vi "GUI_FilterWheels-BellaAlpha.vi"() -> ()   [LabVIEW 2020]
uses:
  Device Drivers/FilterWheels/posTypDef.ctl
  Device Drivers/FilterWheels/ModeTypDEf.ctl
  <vilib>/Utility/file.llb/Read From Spreadsheet File (string).vi
panel:
  out "reference out":refnum<vi>
  out "#ofChannels":i32
  out "indecator ref array":refnum<vi>[](array[refnum])
  in  "time to wait (TCP) 2":i32=10
  in  "plot":bool=TRUE
  out "ratio(h)":bool
  out "fixsize":bool
  in  "shotnumber":i32
  out "error (h)":bool
  out "Device Name (h)":string="StagingDG645 1"
  in  "Main Tap":T1(tab)
  out "LoadOut":string[][](array[string])
  in  "Path":path=path "H:/data/ECS dumps/FilterWheels"
  in  "ModeAll":T2
  in  "modeArray":T2[](array[typedef])
  out "Status 2":u32[](array[colorbox])
  out "Name":string[](array[string])
  in  "pos":T3[](array[typedef])
  out "device status":string
  out "local Port":u16=65427
  out "port or service name":u16=65426
  out "Remote Host":string="192.168.11.97"
  in  "timeout ms (slow resp)":i32=500
  in  "reset":bool
  out "All Devices (h)":string[](array[string])=["StagingDG645 1", "StagingDG645 2"]
  in  "time to wait (TCP)":i32=10
  out "error out":errorcluster
  out "connections (hidden)":variant[](array[variant])=[variant(refnum<k16> refnum), variant(refnum<k16> refnum)]
  in  "time to wait (main loop)":i32=10
  out "Data String":string="Amplitude.Ch AB,3.000000000000\r\nAmplitude.Ch CD,4.000000000000\r\nAmplitude.Ch EF,4.000000000000\r\nAmplitude.Ch GH,4.000000000000\r\nAmplitude.Ch T0,4.000000000000\r\nDelay.Ch A,0.000000000000\r\nDelay.Ch B,0.030000000000\r\nDelay.Ch C,0.000000000000\r\nDelay.Ch D,0.030000000000\r\nDelay.Ch E,0.000000000000\r\nDelay.Ch F,0.030000000000\r\nDelay.Ch G,0.000000000000\r\nDelay.Ch H,0.030000000000\r\nDelay.Ch T0,0.000000000000\r\nDelay.Ch T1,0.030000\r\nInhibit,Triggers\r\nLinked.Ch A,T0\r\nLinked.Ch B,A\r\nLinked.Ch C,T0\r\nLinked.Ch D,C\r\nLinked.Ch E,T0\r\nLinked.Ch F,E\r\nLinked.Ch G,T0\r\nLinked.Ch H,G\r\nLocalSavingPath,c:\\temp\r\nSave,off\r\nTrigger.ExecuteSingleShot,\r\nTrigger.Level,1.000000\r\nTrigger.Rate,10.000000\r\nTrigger.Source,External rising edges\r\ntimeout,0.000000\r\nPolarity.Ch AB,Positive\r\nPolarity.Ch CD,Positive\r\nPolarity.Ch EF,Positive\r\nPolarity.Ch GH,Positive\r\nPolarity.Ch T0,Positive\r\n"
  in  "Local Saving Path":path
  out "concatenated string":string
  out "subscriberString":string
  out "error message":string
  out "new data":bool
  out "Data Connection out":bool=TRUE
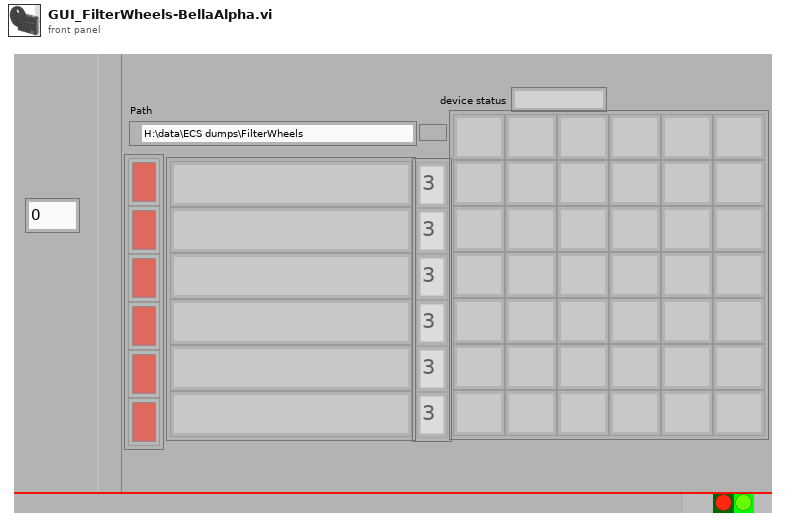
[diagram p1: front panel]
types:
  T1 = enum32{"All Channels", "Network", "Internal", "Advanced"}
  T2 = typedef "ModeTypDEf.ctl" = enum16{"Diode", "Low Power", "High Power", "undefined"}
  T3 = typedef "posTypDef.ctl" = enum16{"1", "2", "3", "4", "5", "6"}
  T4 = typedef "EventTypDef.ctl" = refnum<user-event>
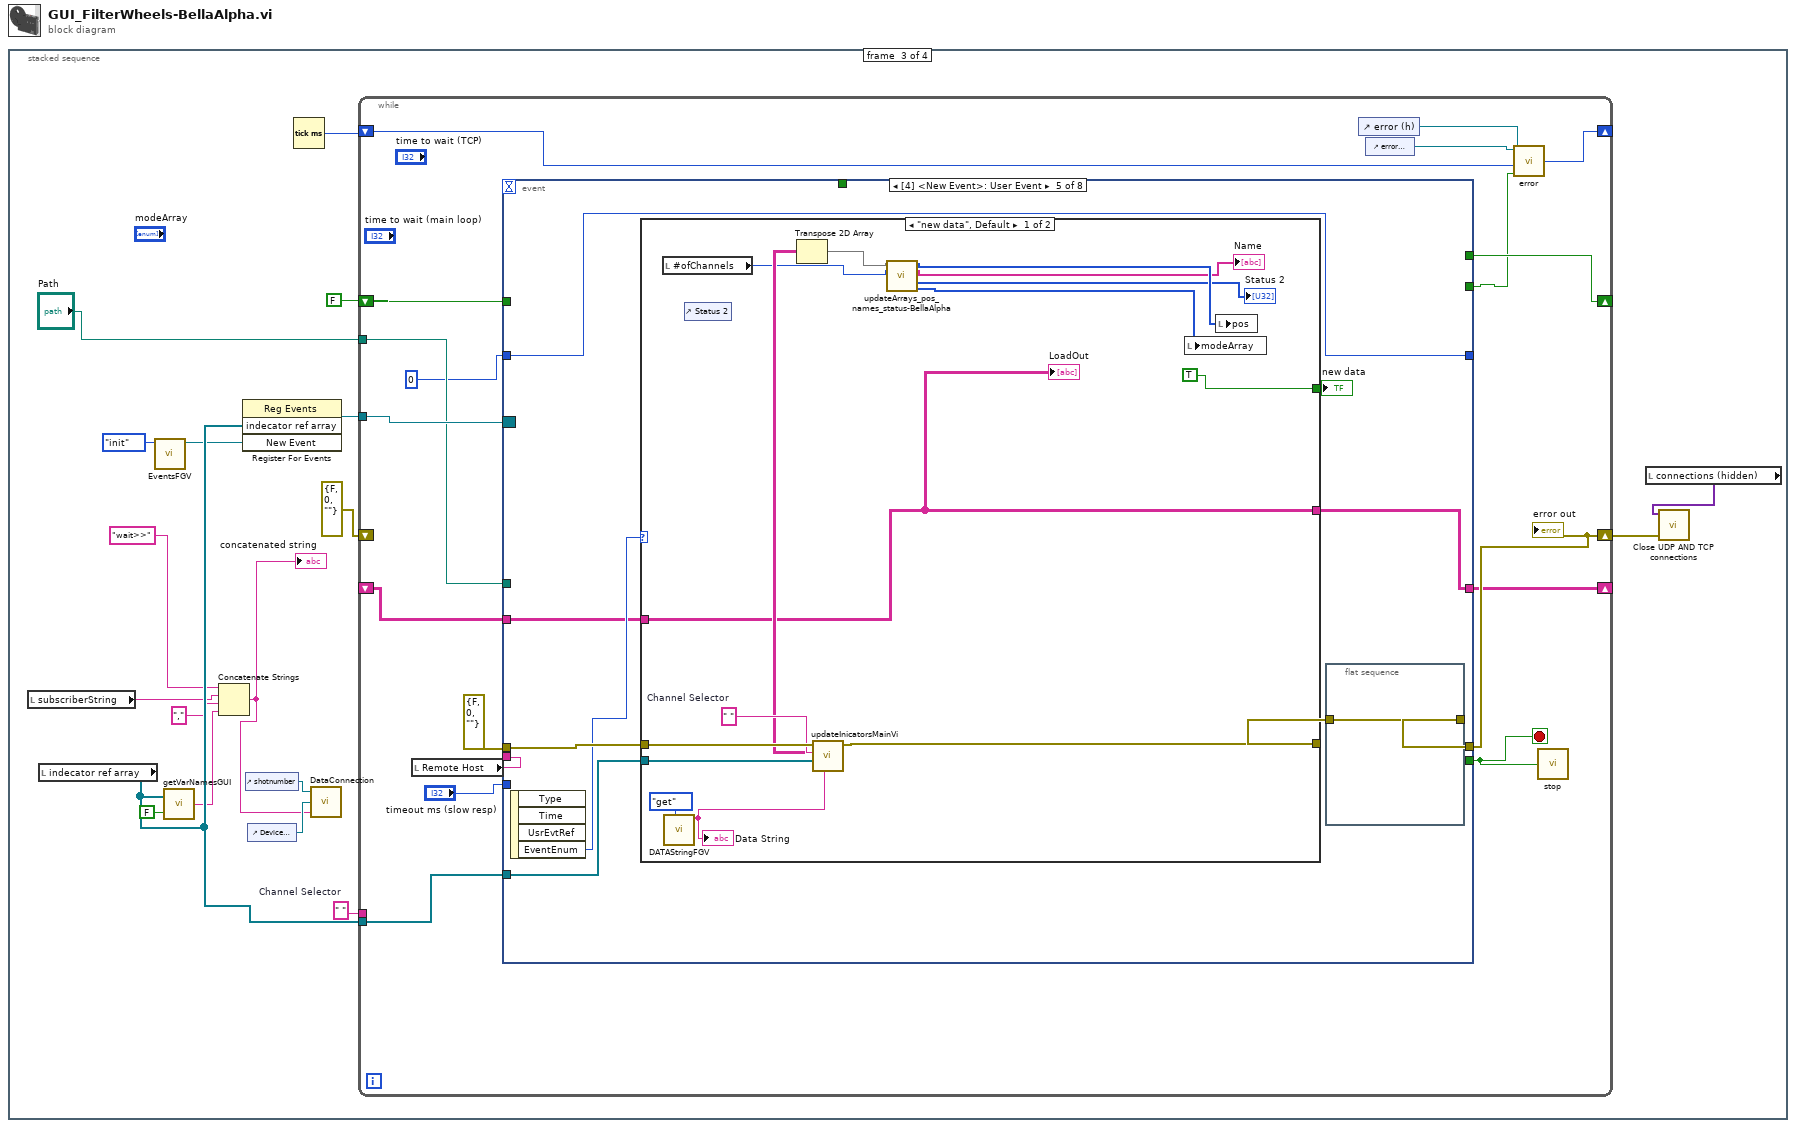
[diagram p0: block diagram]
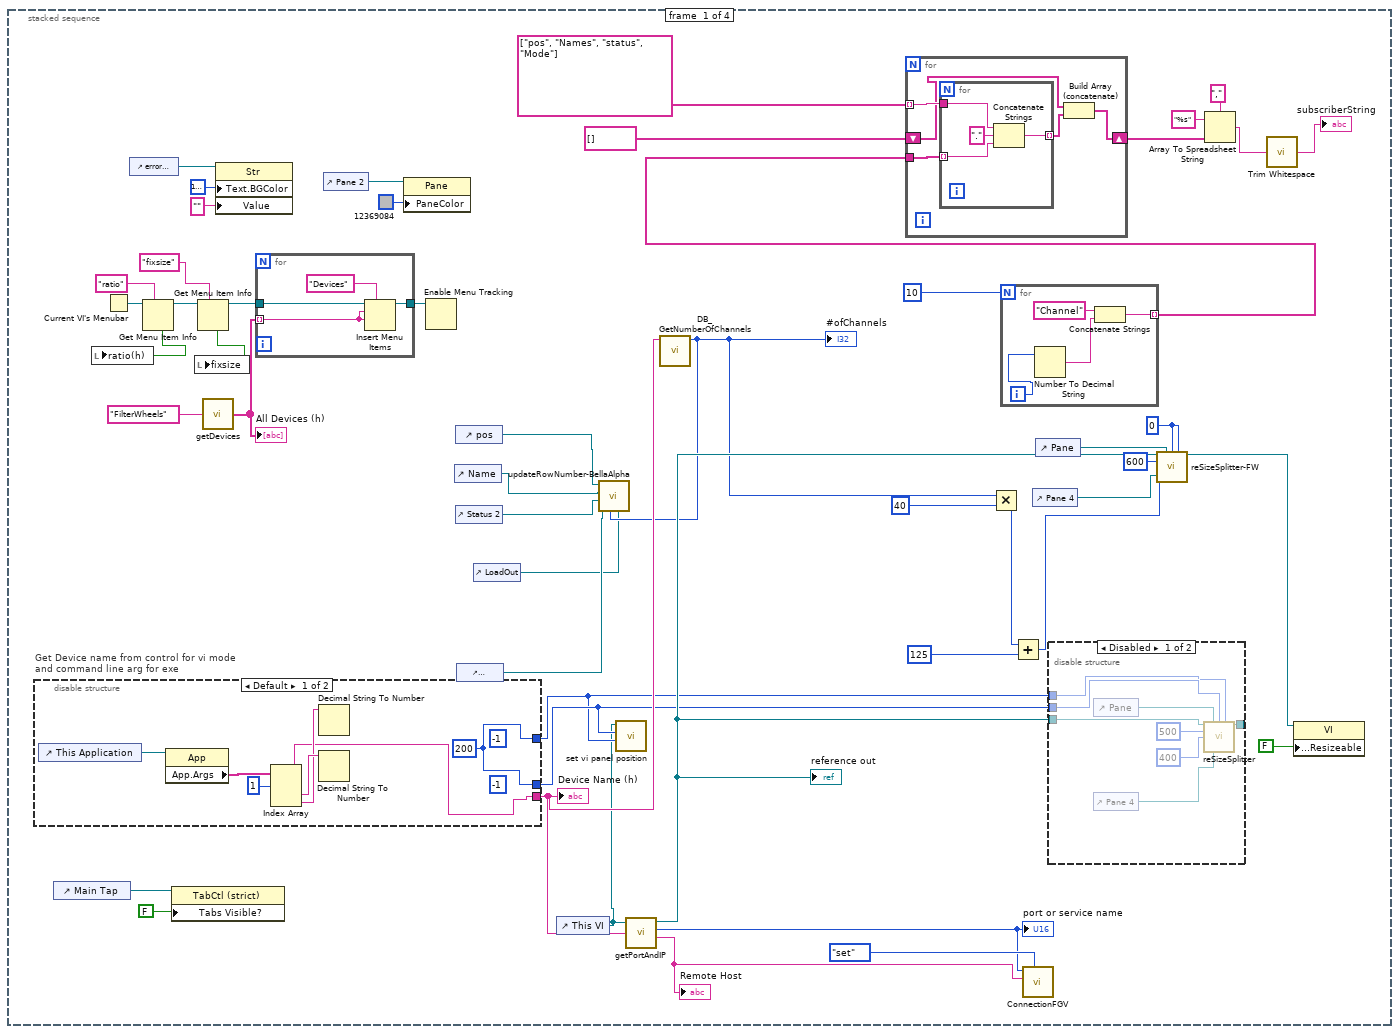
[diagram p2: hidden frame]
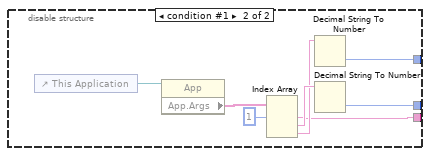
[diagram p4: hidden frame]
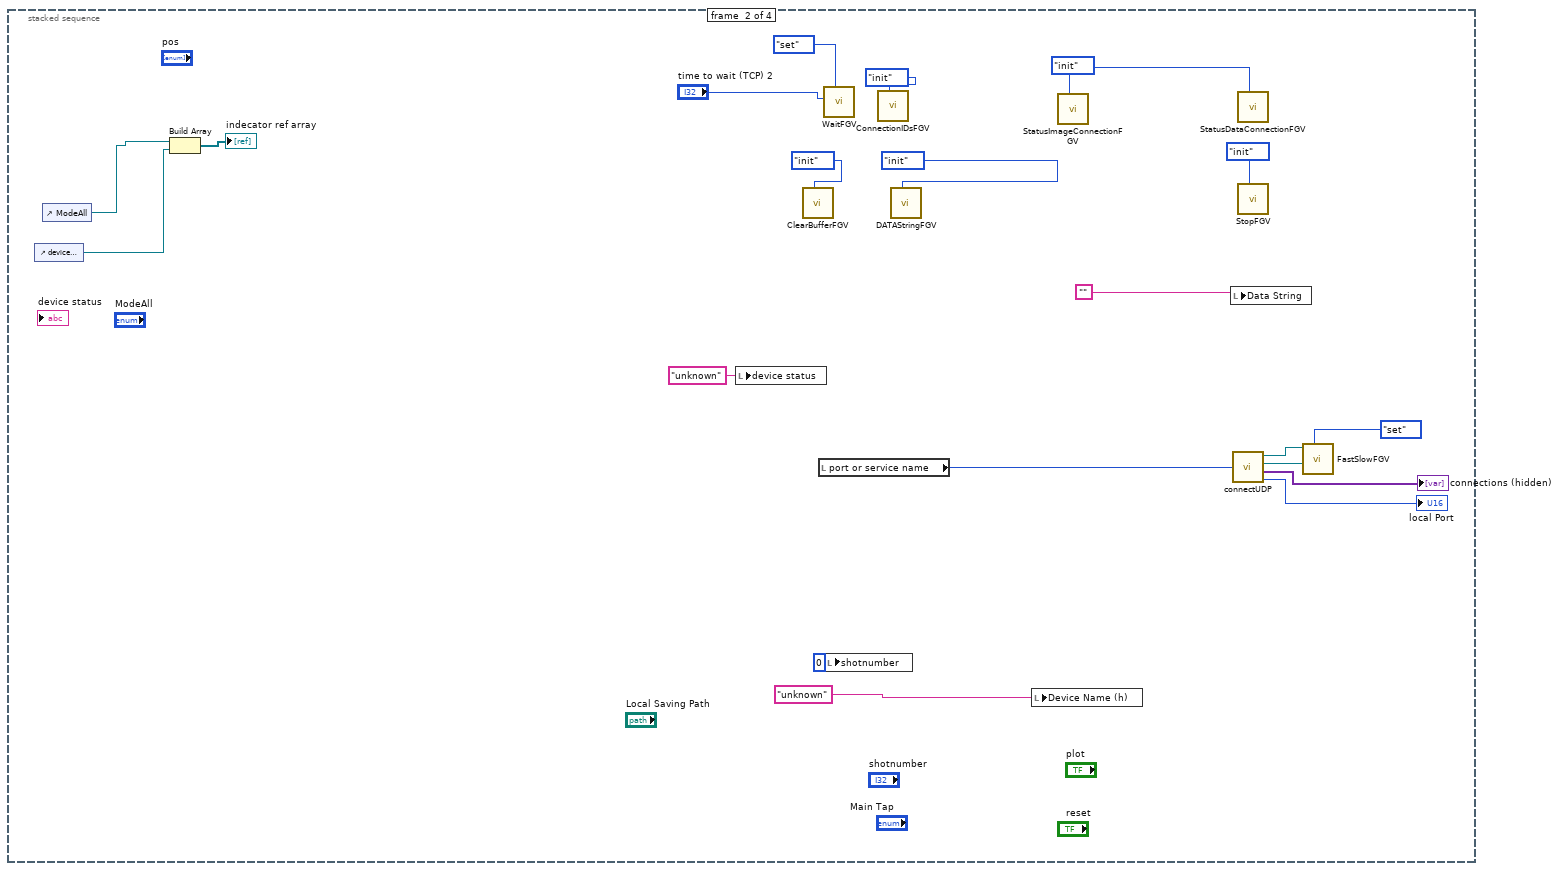
[diagram p5: hidden frame]
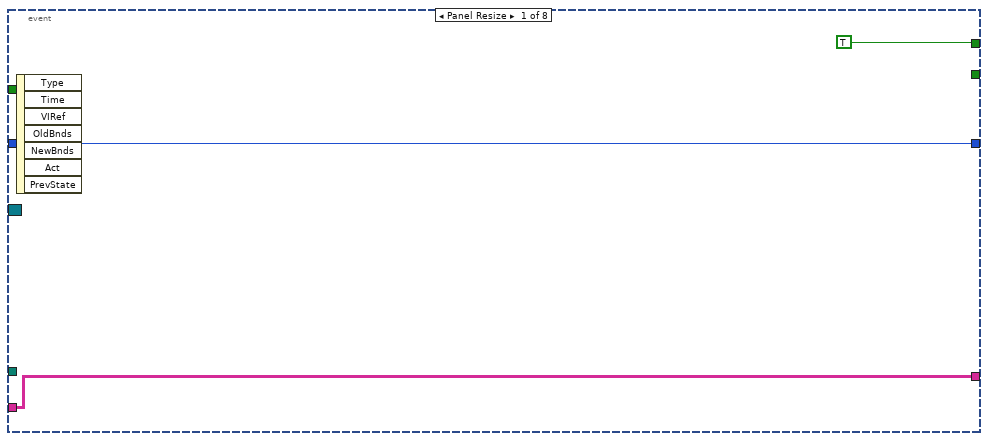
[diagram p6: hidden frame]
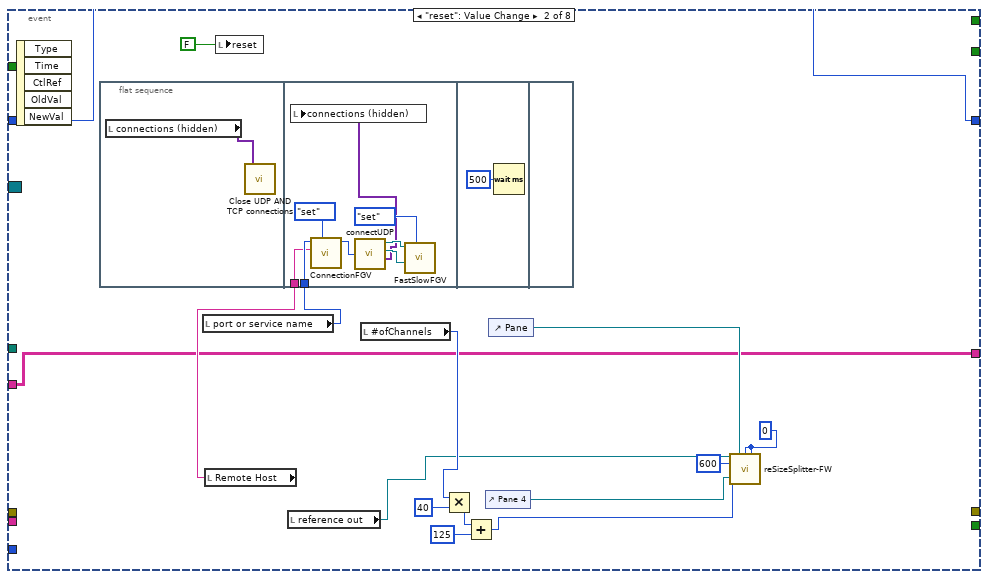
[diagram p7: hidden frame]
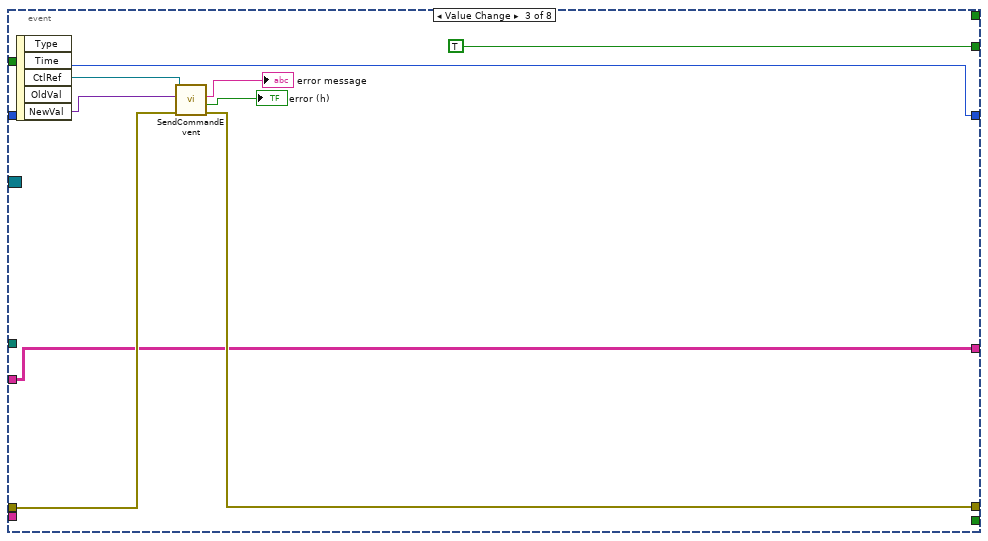
[diagram p8: hidden frame]
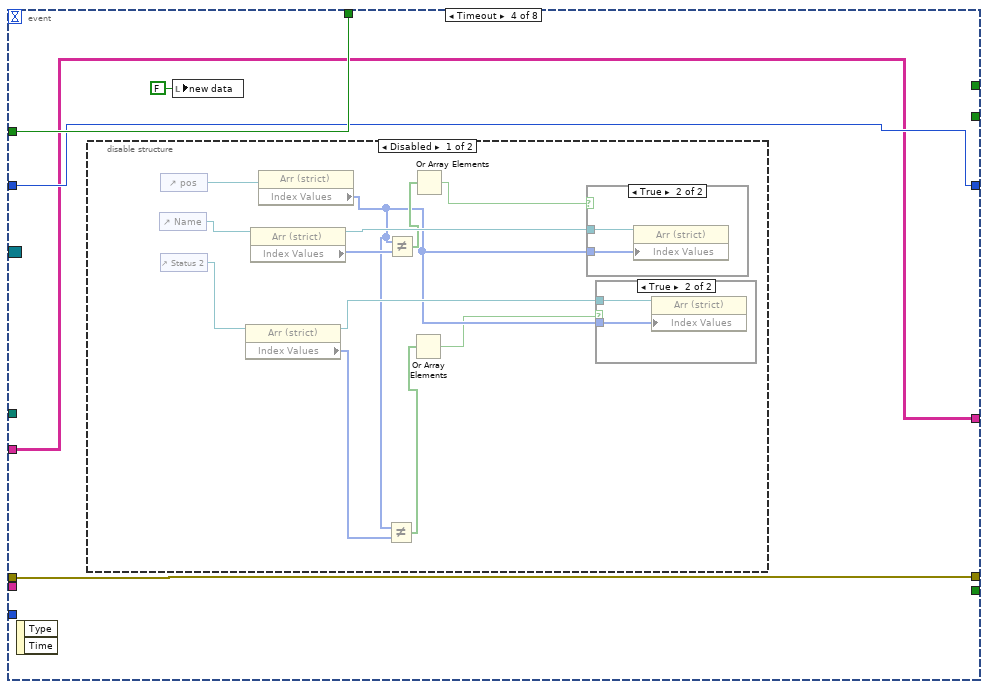
[diagram p9: hidden frame]
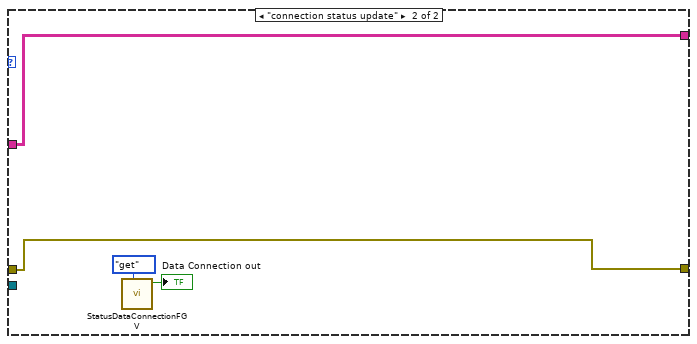
[diagram p13: hidden frame]
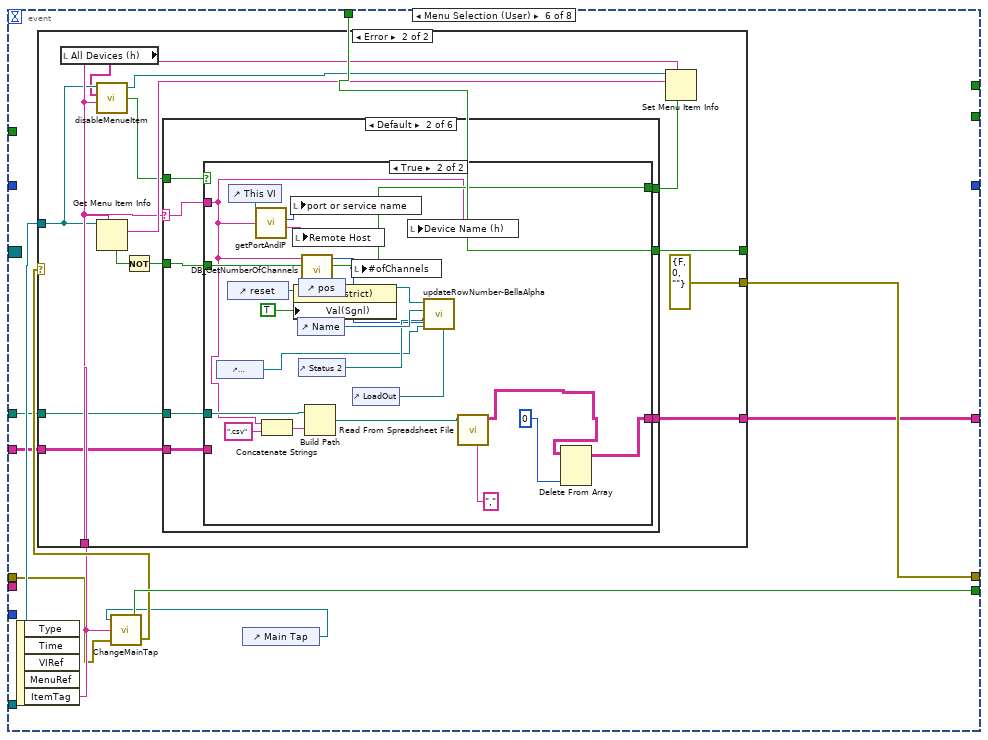
[diagram p14: hidden frame]
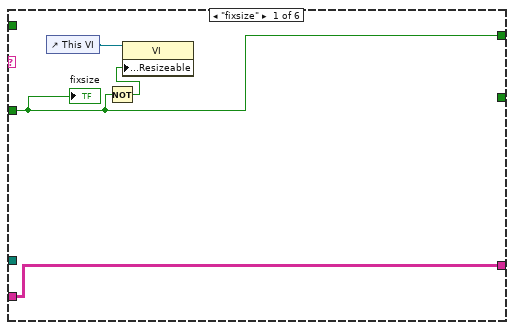
[diagram p16: hidden frame]
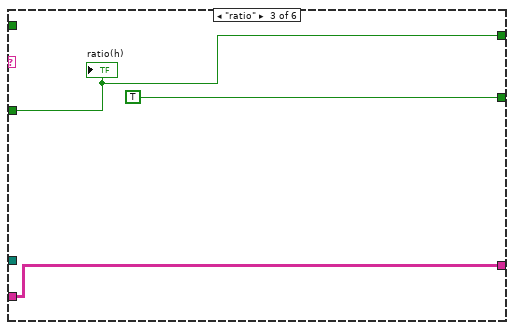
[diagram p18: hidden frame]
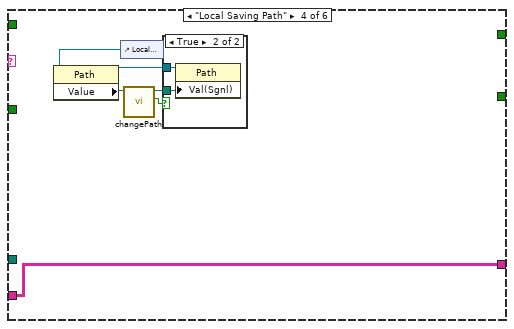
[diagram p19: hidden frame]
diagram:
  n1 = stacked-sequence {
    frame #0 {
      w1 = i16 0 ("top")
      n2 = disable-structure "Get Device name from control for vi mode\nand command line arg for exe" shown="Default" {
        disable-tunnel: [w78 w84] -> w29
        disable-tunnel: [w77 w87] -> w11
        disable-tunnel: [w77 w86] -> w10
        frame condition #0 (active) {
          w77 = i16 200 ("left")
          (unwired) i16 -1 ("left")
          (unwired) i16 -1 ("left")
          n3 = control-ref of="This Application"() -> (w83:refnum<vi>)
          n4 = property class="App"(reference=w83) -> ("App.Args"=w79:string[])  [unwired: 1 in, 2 out]
          n5 = Index Array(array=w79, index #1=1 ("index")) -> (element #1=w78:string, element #2=w81:string, element #3=w80:string)  [unwired: 2 in]
          n6 = Decimal String To Number(string=w80) -> ()  [unwired: 2 in, 2 out]
          n7 = Decimal String To Number(string=w81) -> ()  [unwired: 2 in, 2 out]
        }
        frame condition #1 {
          n8 = control-ref of="This Application"() -> (w91:refnum<vi>)
          n9 = property class="App"(reference=w91) -> ("App.Args"=w85:string[])  [unwired: 1 in, 2 out]
          n10 = Index Array(array=w85, index #1=1 ("index")) -> (element #1=w84:string, element #2=w89:string, element #3=w88:string)  [unwired: 2 in]
          n11 = Decimal String To Number(string=w88) -> (number=w86:i32)  [unwired: 2 in, 1 out]
          n12 = Decimal String To Number(string=w89) -> (number=w87:i32)  [unwired: 2 in, 1 out]
        }
      }
      "Device Name (h)" <- w29
      n13 = control-ref of="Main Tap"() -> (w50:refnum<vi>)
      n14 = Current VI's Menubar() -> (w43:refnum<k9>)
      n15 = control-ref of="error message"() -> (w37:refnum<vi>)
      n16 = Get Menu Item Info(7:"ratio" ("item tag"), 11:w43) -> (3:w41:refnum<k9>, 4:w42:bool)  [unwired: 1 in, 5 out]
      n17 = local write "ratio(h)"(w42) -> ()
      n18 = property class="TabCtl (strict)"(reference=w50, "Tabs Visible?"=FALSE) -> ()  [unwired: 1 in, 2 out]
      n19 = Get Menu Item Info(7:"fixsize" ("item tag"), 11:w41) -> (3:w33:refnum<k9>, 4:w39:bool)  [unwired: 1 in, 5 out]
      n20 = local write "fixsize"(w39) -> ()
      n21 = call "getDevices.vi"("Device Class"="FilterWheels") -> ("All Devices"=w31:string[])
      "All Devices (h)" <- w31
      n22 = property class="Str"(reference=w37, "Text.BGColor"=u32 16777238, "Value"="") -> ()  [unwired: 1 in, 2 out]
      n23 = for {
        tunnel: w33 -> [w67]
        tunnel: [w66] -> w32
        tunnel: w31 -> [w64] mode=indexing
        n24 = Insert Menu Items(5:"Devices" ("menu tag"), 7:w64, 8:w64, 9:w67) -> (3:w66:refnum<k9>)  [unwired: 2 in, 2 out]
      }
      n25 = control-ref of="Pane 2"() -> (w35:refnum<vi>)
      n26 = property class="Pane"(reference=w35, "PaneColor"=u32 12369084) -> ()  [unwired: 1 in, 2 out]
      n27 = Enable Menu Tracking(4:w32) -> ()  [unwired: 2 in, 2 out]
      n28 = control-ref of="Name"() -> (w7:refnum<vi>)
      n29 = control-ref of="pos"() -> (w8:refnum<vi>)
      n30 = control-ref of="Status 2"() -> (w6:refnum<vi>)
      n31 = control-ref of="modeArray"() -> (w5:refnum<vi>)
      n32 = control-ref of="LoadOut"() -> (w3:refnum<vi>)
      n33 = control-ref of="This VI"() -> (w9:refnum<vi>)
      n34 = call "set vi panel position.vi"("top"=w10, "left"=w11, "This VI"=w9) -> ()  [unwired: 7 in, 2 out]
      n35 = call "getPortAndIP.vi"("Device Name"=w29, "This Vi"=w9) -> ("Remote Host"=w46:string, "port or service name"=w45:u16, "reference out"=w18:refnum<vi>)  [unwired: 2 in, 2 out]
      "port or service name" <- w45
      "Remote Host" <- w46
      "reference out" <- w18
      n36 = call "DB_GetNumberOfChannels.vi"("DeviceName"=w29) -> ("Numeric"=w4:i32)  [unwired: 9 in, 1 out]
      "#ofChannels" <- w4
      n37 = call "updateRowNumber-BellaAlpha.vi"("LoadOut"=w3, "Numeric"=w4, "modeArray 2"=w5, "Status 3"=w6, "Name"=w7, "Array in"=w8) -> ()  [unwired: 6 in]
      n38 = Multiply(x=w4, y=40) -> (x*y=w12:i32)
      n39 = for {
        N: 10 -> [_]
        tunnel: [w60] -> w27 mode=indexing
        i -> [w63]
        n40 = Number To Decimal String(number=w63) -> (decimal integer string=w61:string)  [unwired: 1 in]
        n41 = Concatenate Strings("Channel" ("string"), w61) -> (w60:string)
      }
      n42 = for {
        tunnel: string[] ["pos", "Names", "status", "Mode"] -> [w54] mode=indexing
        tunnel: w27 -> [w55]
        shift-right: [w52] -> w24
        shift-left: string[] [] -> [w51]
        n43 = for {
          tunnel: w55 -> [w57] mode=indexing
          tunnel: w54 -> [w59]
          tunnel: [w56] -> w53 mode=indexing
          n44 = Concatenate Strings(w59, "." ("string"), w57) -> (w56:string)
        }
        n45 = Build Array (concatenate)(w51, w53) -> (w52:string[])
      }
      n46 = Add(x=w12, y=125) -> (x+y=w13:i32)
      n47 = call "ConnectionFGV.vi"("command"=enum16{"get", "set", "init"}."set", "Remote Host in"=w46, "port or service name in"=w45) -> ()  [unwired: 7 in, 2 out]
      n48 = control-ref of="Pane 4"() -> (w16:refnum<vi>)
      n49 = control-ref of="Pane"() -> (w19:refnum<vi>)
      n50 = disable-structure shown="Disabled" {
        disable-tunnel: w11 -> [w74 _]
        disable-tunnel: w10 -> [w73 _]
        disable-tunnel: w18 -> [w71 w76]
        disable-tunnel: [w68 w76] -> _
        frame Disabled {
          n51 = control-ref of="Pane"() -> (w75:refnum<vi>)
          n52 = control-ref of="Pane 4"() -> (w72:refnum<vi>)
          n53 = call "reSizeSplitter.vi"("this vi"=w71, "pane"=w75, "left"=w74, "top"=w73, "Width"=u32 500, "Height"=u32 400, "pane2"=w72) -> ("reference out"=w68:refnum<vi>)  [unwired: 8 in]
        }
        frame Enabled {
        }
      }
      n54 = call "reSizeSplitter-FW.vi"("this vi"=w18, "pane"=w19, "left"=w1, "top"=w1, "Width"=u32 600, "Height"=w13, "pane2"=w16) -> ("reference out"=w17:refnum<vi>)  [unwired: 8 in]
      n55 = Array To Spreadsheet String(delimiter (Tab)=",", array=w24, 3:"%s" ("format string")) -> (spreadsheet string=w22:string)
      n56 = call <vilib>:"Trim Whitespace.vi"("string"=w22) -> ("trimmed string"=→"subscriberString":string)  [unwired: 1 in]
      n57 = property class="VI"(reference=w17, "Front Panel.Resizeable"=FALSE ("Front Panel Window:Resizable")) -> ()  [unwired: 1 in, 2 out]
    }
    frame #1 {
      w104 = enum16{"get", "set", "init"}."init" ("Command")
      n58 = control-ref of="device status"() -> (w93:refnum<vi>)
      n59 = control-ref of="ModeAll"() -> (w94:refnum<vi>)
      n60 = Build Array(w94, w93) -> (→"indecator ref array":refnum<vi>[])
      n61 = local write "device status"("unknown" ("device status")) -> ()
      n62 = call "ClearBufferFGV.vi"("Command"=enum16{"set", "get", "init"}."init") -> ()  [unwired: 10 in, 1 out]
      n63 = local read "port or service name"() -> (w100:u16)
      n64 = call "WaitFGV.vi"("Command"=enum16{"get", "set", "init"}."set", "milliseconds to wait"="time to wait (TCP) 2") -> ()  [unwired: 9 in, 1 out]
      n65 = local write "shotnumber"(0 ("shotnumber")) -> ()
      n66 = call "ConnectionIDsFGV.vi"("Command"=enum16{"add", "get", "init"}."init") -> ()  [unwired: 10 in, 1 out]
      n67 = call "DATAStringFGV.vi"("Command"=enum16{"get", "set", "init"}."init") -> ()  [unwired: 9 in, 2 out]
      n68 = local write "Device Name (h)"("unknown" ("Device Name")) -> ()
      n69 = call "StatusImageConnectionFGV.vi"("Command"=w104) -> ()  [unwired: 10 in, 1 out]
      n70 = local write "Data String"("") -> ()
      n71 = call "connectUDP.vi"("port or service name NOT USED"=w100) -> ("fast ID (h)"=w99:refnum<k16>, "slow ID (h)"=w98:refnum<k16>, "connections (hidden)"=→"connections (hidden)":variant[], "local Port"=→"local Port":u16)
      n72 = call "StatusDataConnectionFGV.vi"("Command"=w104) -> ()  [unwired: 10 in, 1 out]
      n73 = call "StopFGV.vi"("Command"=enum16{"set", "get", "init"}."init") -> ()  [unwired: 9 in, 2 out]
      n74 = call "FastSlowFGV.vi"("Command"=enum16{"get", "set", "init"}."set", "slow ID"=w98, "fast ID"=w99) -> ()  [unwired: 7 in, 2 out]
    }
    frame #2 {
      w122 = " "  # Channel Selector
      n75 = local read "subscriberString"() -> (w117:string)
      n76 = local read "indecator ref array"() -> (w121:refnum<vi>[])
      n77 = call "EventsFGV.vi"("Command"=enum16{"get", "init"}."init") -> ("New Event"=w114:T4)  [unwired: 9 in, 1 out]
      n78 = call "getVarNamesGUI.vi"("start"=FALSE, "Array"=w121) -> ("String"=w116:string)
      n79 = Concatenate Strings("wait>>" ("string"), w117, "," ("string"), w116) -> (w119:string)
      "concatenated string" <- w119
      n80 = register-events(w121, w114) -> (reference out=w123:refnum<event-registration>)  [unwired: 2 in, 1 out]
      n81 = control-ref of="shotnumber"() -> (w125:refnum<vi>)
      n82 = control-ref of="Device Name (h)"() -> (w124:refnum<vi>)
      n83 = Tick Count (ms)() -> (millisecond timer value=w126:u32)
      n84 = call "DataConnection.vi"("Subscriber list"=w119, "Device Name (h)"=w124, "shotnumber"=w125) -> ()
      n85 = while {
        shift-right: [w136] -> w129
        shift-left: errorcluster {"status"=FALSE, "code"=0, "source"=""} ("error out") -> [_]
        tunnel: w121 -> [w137]
        shift-right: [w145] -> _
        shift-left: FALSE -> [w146]
        shift-right: [w144] -> _
        shift-left: w126 -> [w143]
        tunnel: w123 -> [w141]
        tunnel: w122 -> [_]
        tunnel: "Path" -> [w134]
        shift-right: [w132] -> _
        shift-left: _ -> [w131]
        stop <- w142 stop-if-true
        n86 = local read "Remote Host"() -> (w147:string)
        n87 = event shown="[4] <New Event>: User Event" {
          selector: w141 -> [_ _ _ _ _ _ _ _]
          dyn-events: _ -> [_ _ _ _ _ _ _ _]
          timeout: _ -> [_ _ _ _ _ _ _ _]
          tunnel: [_ _ w183 w190 w212 w240 w318 w344] -> w136
          tunnel: w147 -> [_ _ _ _ _ _ _ _]
          tunnel: "timeout ms (slow resp)" -> [_ _ _ _ _ _ _ _]
          tunnel: errorcluster {"status"=FALSE, "code"=0, "source"=""} ("error out") -> [_ _ w180 w190 w215 w241 w318 w344]
          tunnel: [_ _ TRUE _ _ _ TRUE TRUE] -> w135
          tunnel: [_ _ _ _ _ w246 _ _] -> w142
          tunnel: [_ _ _ w189 _ w243 _ _] -> _
          tunnel: w146 -> [_ _ _ w189 _ _ _ _]
          tunnel: [TRUE _ _ _ _ _ _ _] -> w145
          tunnel: w137 -> [_ _ _ _ w214 _ _ _]
          tunnel: 0 -> [w150 w155 w178 w187 w209 _ w314 w338]
          tunnel: [w150 w155 w178 w187 w209 _ w314 w338] -> _
          tunnel: w134 -> [_ _ _ _ _ w238 _ _]
          tunnel: [w149 w154 w177 w186 w207 w237 w313 w337] -> w132
          tunnel: w131 -> [w149 w154 w177 w186 w208 w236 w313 w337]
          event Panel Resize {
            n88 = event-data() -> ()  [unwired: 1 in, 7 out]
          }
          event "reset": Value Change {
            w152 = i16 0 ("top")
            n89 = event-data() -> ()  [unwired: 1 in, 5 out]
            n90 = flat-sequence {
              tunnel: w165 -> [w170]
              tunnel: w164 -> [w169]
              frame #0 {
                n91 = local read "connections (hidden)"() -> (w167:variant[])
                n92 = call "Close UDP AND TCP connections.vi"("appended array"=w167) -> ()  [unwired: 7 in]
              }
              frame #1 {
                n93 = call "ConnectionFGV.vi"("command"=enum16{"get", "set", "init"}."set", "Remote Host in"=w169, "port or service name in"=w170) -> ("port or service name out"=w174:u16)  [unwired: 7 in, 1 out]
                n94 = call "connectUDP.vi"("port or service name NOT USED"=w174) -> ("fast ID (h)"=w173:refnum<k16>, "slow ID (h)"=w172:refnum<k16>, "connections (hidden)"=w168:variant[])  [unwired: 1 out]
                n95 = local write "connections (hidden)"(w168) -> ()
                n96 = call "FastSlowFGV.vi"("Command"=enum16{"get", "set", "init"}."set", "slow ID"=w172, "fast ID"=w173) -> ()  [unwired: 7 in, 2 out]
              }
              frame #2 {
                n97 = Wait (ms)(milliseconds to wait=u32 500) -> ()  [unwired: 1 out]
              }
              frame #3 {
              }
            }
            n98 = local read "port or service name"() -> (w165:u16)
            n99 = local read "Remote Host"() -> (w164:string)
            n100 = local write "reset"(FALSE ("reset")) -> ()
            n101 = local read "reference out"() -> (w156:refnum<vi>)
            n102 = local read "#ofChannels"() -> (w157:i32)
            n103 = Multiply(x=w157, y=40) -> (x*y=w163:i32)
            n104 = Add(x=w163, y=125) -> (x+y=w162:i32)
            n105 = control-ref of="Pane 4"() -> (w159:refnum<vi>)
            n106 = control-ref of="Pane"() -> (w158:refnum<vi>)
            n107 = call "reSizeSplitter-FW.vi"("this vi"=w156, "pane"=w158, "left"=w152, "top"=w152, "Width"=u32 600, "Height"=w162, "pane2"=w159) -> ()  [unwired: 8 in, 1 out]
          }
          event Value Change {
            n108 = event-data() -> ("CtlRef"=w185:refnum<vi>, "NewVal"=w184:variant)  [unwired: 1 in, 3 out]
            n109 = call "SendCommandEvent.vi"("error out 2"=w180, "NewVal"=w184, "CtlRef"=w185) -> ("error out"=w183:errorcluster, "error (h)"=→"error (h)":bool, "error message"=→"error message":string)  [unwired: 5 in, 1 out]
          }
          event Timeout {
            n110 = event-data() -> ()  [unwired: 1 in, 2 out]
            n111 = disable-structure shown="Disabled" {
              frame Disabled {
                n112 = control-ref of="Name"() -> (w199:refnum<vi>)
                n113 = control-ref of="pos"() -> (w202:refnum<vi>)
                n114 = control-ref of="Status 2"() -> (w201:refnum<vi>)
                n115 = property class="Arr (strict)"(reference=w201) -> (reference out=w200:refnum<vi>, "Index Values"=w193:u32[])  [unwired: 1 in, 1 out]
                n116 = property class="Arr (strict)"(reference=w199) -> (reference out=w198:refnum<vi>, "Index Values"=w197:u32[])  [unwired: 1 in, 1 out]
                n117 = property class="Arr (strict)"(reference=w202) -> ("Index Values"=w192:u32[])  [unwired: 1 in, 2 out]
                n118 = Not Equal?(x=w192, y=w193) -> (x != y?=w194:bool[])
                n119 = Not Equal?(x=w192, y=w197) -> (x != y?=w196:bool[])
                n120 = Or Array Elements(Boolean array=w194) -> (logical OR=w191:bool)
                n121 = Or Array Elements(Boolean array=w196) -> (logical OR=w195:bool)
                n122 = case shown="True" w195 {
                  tunnel: w198 -> [_ w206]
                  tunnel: w192 -> [_ w205]
                  frame False {
                  }
                  frame True {
                    n123 = property class="Arr (strict)"(reference=w206, "Index Values"=w205) -> ()  [unwired: 1 in, 2 out]
                  }
                }
                n124 = case shown="True" w191 {
                  tunnel: w200 -> [_ w204]
                  tunnel: w192 -> [_ w203]
                  frame False {
                  }
                  frame True {
                    n125 = property class="Arr (strict)"(reference=w204, "Index Values"=w203) -> ()  [unwired: 1 in, 2 out]
                  }
                }
              }
              frame Enabled {
              }
            }
            n126 = local write "new data"(FALSE ("new data")) -> ()
          }
          event User Event {
            n127 = event-data() -> ("EventEnum"=w211:enum16{"new data", "connection status update"})  [unwired: 1 in, 3 out]
            n128 = case shown="\"new data\", Default" w211 {
              tunnel: w215 -> [w231 w233]
              tunnel: [w230 w233] -> w213
              tunnel: w214 -> [w228 _]
              tunnel: [TRUE ("new data") _] -> w210
              tunnel: w208 -> [w217 w232]
              tunnel: [w217 w232] -> w207
              frame "new data", Default {
                w229 = " "  # Channel Selector
                n129 = local read "#ofChannels"() -> (w222:i32)
                n130 = call "DATAStringFGV.vi"("Command"=enum16{"get", "set", "init"}."get") -> ("Data String out"=w226:string)  [unwired: 9 in, 1 out]
                "Data String" <- w226
                n131 = control-ref of="Status 2"() -> ()  [unwired: 1 out]
                n132 = call "updateInicatorsMainVi.vi"("Data String out"=w226, "Array"=w228, "Channel Selector"=w229, "error in"=w231) -> ("name/data"=w225:string[][], "error out"=w230:errorcluster)  [unwired: 5 in, 1 out]
                n133 = Transpose 2D Array(2D array=w225) -> (transposed array=w223:string[][])
                n134 = call "updateArrays_pos_names_status-BellaAlpha.vi"("name/data 2"=w223, "#ofChannels"=w222) -> ("pos"=w221:T3[], "Names"=→"Name":string[], "Status"=→"Status 2":u32[], "Mode"=w218:T2[])  [unwired: 9 in, 1 out]
                n135 = local write "modeArray"(w218) -> ()
                n136 = local write "pos"(w221) -> ()
                "LoadOut" <- w217
              }
              frame "connection status update" {
                n137 = call "StatusDataConnectionFGV.vi"("Command"=enum16{"get", "set", "init"}."get") -> ("Data Connection out"=→"Data Connection out":bool)  [unwired: 10 in]
              }
            }
            "new data" <- w210
            n138 = flat-sequence {
              tunnel: w213 -> [w216]
              tunnel: [w216] -> w212
              frame #0 {
              }
            }
          }
          event Menu Selection (User) {
            n139 = event-data() -> ("MenuRef"=w242:refnum<k9>, "ItemTag"=w244:string)  [unwired: 1 in, 3 out]
            n140 = control-ref of="Main Tap"() -> (w239:refnum<vi>)
            n141 = call "ChangeMainTap.vi"("error in"=w241, "ItemTag"=w244, "reference"=w239) -> ("error out"=w245:errorcluster, "Boolean"=w246:bool)
            n142 = case shown="Error" w245 {
              selector: w245 -> [w248 _]
              tunnel: w242 -> [_ w257]
              tunnel: [_ w259] -> w243
              tunnel: w244 -> [_ w258]
              tunnel: [w248 errorcluster {"status"=FALSE, "code"=0, "source"=""} ("error IO")] -> w240
              tunnel: w238 -> [_ w251]
              tunnel: [w247 w250] -> w237
              tunnel: w236 -> [w247 w249]
              frame No Error {
              }
              frame Error {
                n143 = local read "All Devices (h)"() -> (w252:string[])
                n144 = call "disableMenueItem.vi"("ItemTag"=w258, "All Devices (h)"=w252, "MenuRef"=w257) -> ("this is a Device(tag)"=w256:bool, "menu reference out"=w255:refnum<k9>)  [unwired: 1 in, 1 out]
                n145 = Get Menu Item Info(7:w258, 11:w257) -> (2:w261:string, 4:w262:bool)  [unwired: 1 in, 5 out]
                n146 = Not(x=w262) -> (.not. x?=w260:bool)
                n147 = case shown="Default" w258 {
                  selector: w258 -> [_ w272 _ _ _ _]
                  tunnel: w260 -> [w264 w270 w297 _ _ _]
                  tunnel: [_ _ TRUE _ _ _] -> w259
                  tunnel: w256 -> [_ w273 _ _ _ _]
                  tunnel: [w264 w271 w297 _ _ _] -> w254
                  tunnel: w251 -> [_ w269 _ _ _ _]
                  tunnel: [w263 w268 w296 w299 w307 w310] -> w250
                  tunnel: w249 -> [w263 w267 w296 w299 w307 w310]
                  frame "fixsize" {
                    n148 = control-ref of="This VI"() -> (w266:refnum<vi>)
                    n149 = Not(x=w264) -> (.not. x?=w265:bool)
                    n150 = property class="VI"(reference=w266, "Front Panel.Resizeable"=w265) -> ()  [unwired: 1 in, 2 out]
                    "fixsize" <- w264
                  }
                  frame Default {
                    n151 = case shown="True" w273 {
                      tunnel: w272 -> [_ w286]
                      tunnel: [_ w290] -> w271
                      tunnel: w270 -> [_ w290]
                      tunnel: w269 -> [_ w289]
                      tunnel: [w274 w276] -> w268
                      tunnel: w267 -> [w274 _]
                      frame False {
                      }
                      frame True {
                        n152 = control-ref of="modeArray"() -> (w280:refnum<vi>)
                        n153 = control-ref of="reset"() -> (w292:refnum<vi>)
                        n154 = control-ref of="This VI"() -> (w295:refnum<vi>)
                        n155 = call "getPortAndIP.vi"("Device Name"=w286, "This Vi"=w295) -> ("Remote Host"=w294:string, "port or service name"=w293:u16)  [unwired: 2 in, 3 out]
                        n156 = Concatenate Strings(w286, ".csv" ("string")) -> (w288:string)
                        n157 = local write "port or service name"(w293) -> ()
                        n158 = local write "Remote Host"(w294) -> ()
                        n159 = property class="Bool (strict)"(reference=w292, "Val(Sgnl)"=TRUE ("Value (Signaling)")) -> ()  [unwired: 1 in, 2 out]
                        n160 = control-ref of="Name"() -> (w282:refnum<vi>)
                        n161 = control-ref of="pos"() -> (w283:refnum<vi>)
                        n162 = control-ref of="Status 2"() -> (w281:refnum<vi>)
                        n163 = call "DB_GetNumberOfChannels.vi"("DeviceName"=w286) -> ("Numeric"=w278:i32)  [unwired: 9 in, 1 out]
                        n164 = Build Path(base path=w289, name or relative path=w288) -> (appended path=w285:path)
                        n165 = local write "#ofChannels"(w278) -> ()
                        n166 = control-ref of="LoadOut"() -> (w279:refnum<vi>)
                        n167 = local write "Device Name (h)"(w286) -> ()
                        n168 = call "updateRowNumber-BellaAlpha.vi"("LoadOut"=w279, "Numeric"=w278, "modeArray 2"=w280, "Status 3"=w281, "Name"=w282, "Array in"=w283) -> ()  [unwired: 6 in]
                        n169 = call-poly <vilib>:"Read From Spreadsheet File.vi"("delimiter (\\t)"="," ("delimiter (\\t)"), "file path (dialog if empty)"=w285) -> ("all rows"=w275:string[][])  [unwired: 5 in, 4 out]
                        n170 = Delete From Array(array=w275, index (col)=0 ("disabled index (col)")) -> (array with subset deleted=w276:string[][])  [unwired: 2 in, 1 out]
                      }
                    }
                  }
                  frame "ratio" {
                    "ratio(h)" <- w297
                  }
                  frame "Local Saving Path" {
                    n171 = control-ref of="Local Saving Path"() -> (w300:refnum<vi>)
                    n172 = property class="Path"(reference=w300) -> (reference out=w303:refnum<vi>, "Value"=w304:path)  [unwired: 1 in, 1 out]
                    n173 = call "changePath.vi"("Local Saving in (h)"=w304) -> ("change (h)"=w302:bool, "Local Saving out (h)"=w301:path)  [unwired: 9 in]
                    n174 = case shown="True" w302 {
                      tunnel: w303 -> [_ w306]
                      tunnel: w301 -> [_ w305]
                      frame False {
                      }
                      frame True {
                        n175 = property class="Path"(reference=w306, "Val(Sgnl)"=w305) -> ()  [unwired: 1 in, 2 out]
                      }
                    }
                  }
                  frame "reset" {
                    n176 = control-ref of="reset"() -> (w309:refnum<vi>)
                    n177 = property class="Bool (strict)"(reference=w309, "Val(Sgnl)"=TRUE ("Value (Signaling)")) -> ()  [unwired: 1 in, 2 out]
                  }
                  frame "clear" {
                    n178 = control-ref of="reset"() -> (w312:refnum<vi>)
                    n179 = property class="Bool (strict)"(reference=w312, "Val(Sgnl)"=TRUE ("Value (Signaling)")) -> ()  [unwired: 1 in, 2 out]
                  }
                }
                n180 = Set Menu Item Info(6:w254, 7:w258, 10:w261, 11:w255) -> ()  [unwired: 3 in, 2 out]
              }
            }
          }
          event "pos": Value Change {
            n181 = event-data() -> ("OldVal"=w336:T3[], "NewVal"=w333:T3[])  [unwired: 1 in, 3 out]
            n182 = Not Equal?(x=w336, y=w333) -> (x != y?=w335:bool[])
            n183 = Search 1D Array(1D array=w335, element=TRUE) -> (index of element=w326:i32)  [unwired: 1 in]
            n184 = Number To Decimal String(number=w326) -> (decimal integer string=w325:string)  [unwired: 1 in]
            n185 = Index Array(array=w333, index=w326) -> (element=w316:T3)
            n186 = To Long Integer(number=w316) -> (32bit integer=w315:i32)
            n187 = call "ConnectionFGV.vi"("command"=enum16{"get", "set", "init"}."get") -> ("Remote Host out"=w331:string, "port or service name out"=w332:u16)  [unwired: 9 in]
            n188 = Increment(x=w315) -> (x+1=w319:i32)
            n189 = Number To Decimal String(number=w319) -> (decimal integer string=w323:string)  [unwired: 1 in]
            n190 = Concatenate Strings("set", "pos.Channel" ("string"), w325, ">>" ("string"), w323) -> (w329:string)
            n191 = call "sendCommandAndListen.vi"("command in"=w329, "error in"=w318, "Remote Host"=w331, "port or service name"=w332) -> ("error"=w321:bool, "error message"=w322:string, "error out"=w320:errorcluster)  [unwired: 8 in, 5 out]
            n192 = local write "error message"(w322) -> ()
            n193 = call <vilib>:"Clear Errors.vi"("error in (no error)"=w320) -> ()  [unwired: 5 in, 2 out]
            n194 = local write "error (h)"(w321) -> ()
          }
          event "modeArray": Value Change {
            n195 = event-data() -> ("OldVal"=w360:T2[], "NewVal"=w357:T2[])  [unwired: 1 in, 3 out]
            n196 = Not Equal?(x=w360, y=w357) -> (x != y?=w359:bool[])
            n197 = Search 1D Array(1D array=w359, element=TRUE) -> (index of element=w350:i32)  [unwired: 1 in]
            n198 = Number To Decimal String(number=w350) -> (decimal integer string=w349:string)  [unwired: 1 in]
            n199 = Index Array(array=w357, index=w350) -> (element=w341:T2)
            n200 = call "ConnectionFGV.vi"("command"=enum16{"get", "set", "init"}."get") -> ("Remote Host out"=w355:string, "port or service name out"=w356:u16)  [unwired: 9 in]
            n201 = call <userlib>:"Get Strings from Enum__ogtk.vi"("Enum"=ModeTypDEf."Low Power" ("Mode")) -> ("Enum Strings"=w342:string[])  [unwired: 7 in, 3 out]
            n202 = Index Array(array=w342, index=w341) -> (element=w340:string)
            n203 = Concatenate Strings("set", "Mode.Channel" ("string"), w349, ">>" ("string"), w340) -> (w353:string)
            n204 = call "sendCommandAndListen.vi"("command in"=w353, "error in"=w344, "Remote Host"=w355, "port or service name"=w356) -> ("error"=w346:bool, "error message"=w347:string, "error out"=w345:errorcluster)  [unwired: 8 in, 5 out]
            n205 = local write "error message"(w347) -> ()
            n206 = call <vilib>:"Clear Errors.vi"("error in (no error)"=w345) -> ()  [unwired: 5 in, 2 out]
            n207 = local write "error (h)"(w346) -> ()
          }
        }
        "error out" <- w136
        n208 = control-ref of="error (h)"() -> (w138:refnum<vi>)
        n209 = control-ref of="error message"() -> (w139:refnum<vi>)
        n210 = call "error.vi"("Boolean"=w135, "millisecond timer value"=w143, "reference"=w138, "error message"=w139) -> ("millisecond timer value 2"=w144:u32)
        n211 = call "stop.vi"("Boolean"=w142) -> ()
      }
      n212 = local read "connections (hidden)"() -> (w128:variant[])
      n213 = call "Close UDP AND TCP connections.vi"("error in"=w129, "appended array"=w128) -> ()  [unwired: 6 in]
    }
    frame #3 {
      n214 = control-ref of="Main  Control"() -> (w362:refnum<vi>)
      n215 = property class="TabCtl (strict)"(reference=w362, "Tabs Visible?"=TRUE) -> ()  [unwired: 1 in, 2 out]
      n216 = property class="TabCtl (strict)"(reference=w362, "Tab Location"=enum32{"Top", "Bottom", "Left", "Right"}."Bottom") -> ()  [unwired: 1 in, 2 out]
      n217 = flat-sequence {
        frame #0 {
          n218 = Wait (ms)(milliseconds to wait=u32 0) -> ()  [unwired: 1 out]
        }
        frame #1 {
        }
        frame #2 {
          n219 = control-ref of="This VI"() -> (w367:refnum<vi>)
          n220 = case shown="True" FALSE {
            tunnel: w367 -> [w368 w371]
            tunnel: [w368 w369] -> w366
            frame False {
            }
            frame True {
              n221 = property class="VI" props=["Front Panel.Open"](reference=w371) -> (reference out=w370:refnum<vi>)  [unwired: 1 in, 2 out]
              n222 = invoke class="VI" method="FP.Close"(reference=w370) -> (reference out=w369:refnum<vi>)  [unwired: 2 in, 2 out]
            }
          }
          n223 = Close Reference(reference=w366) -> ()  [unwired: 1 in, 1 out]
        }
      }
    }
  }
